vi "CRYOpen Edit Dialog.vi"(9 "List Index":i32, 10 "Stimulus In":T1={"StimulusType"="", "UseMLValArray"=[], "ML_axisArray"=[], "MLValLevelNameArray"=[], "Level(U)Array"=[1.0, 0.0, 0.0, 0.0, 0.0, 0.0, 0.26], "Start(Stop)FreqArray"=[20000.0, 20.0], "Start(Stop)AmpArray"=[0.5, 1.0], "StepResolutionArray"=[], "Unit_Array"=[], "DegValArray"=[], "DegUnitArray"=[], "Steps1"=19, "Cycle/step1(#)"=20, "Time/step1(s)"=0.01, "Transition1"=0.0, "SweepRate2"=1.0, "Freq3(Hz)"=0.0, "Steps3(#)"=19.0, "Cycles3(#)"=12, "StepSize3"=0.0, "wave time"="", "RMS_Value4"=0.0, "Peak_Value4"=0.0, "WavePath4"="", "RMS_unit4"="", "Peak_unit4"="", "wave Info"="", "dc_ctrl5_1"=0, "dc_ctrl5_2"=0, "dc_polar5"=0, "Max.Current"=0, "Steps5(#)"=19, "Time/Step5"=0.05, "Level5"=0.0, "StepsSize5Val"=0.0, "StepSize5Unit"="", "SweepType"=0, "Fixed/Ratio6"=0, "Transition6"=0.0, "Steps6(#)"=19.0, "Cycle/Steps6(#)"=12, "Time/Steps6(s)"=0.0, "Freq6(Hz)"=0.0, "Difference6(Hz)"=0.0, "Ratio6"="", "NoiseType7"=0, "Duration7(s)"=1.0, "MinFreq7(Hz)"=20000.0, "MaxFreq7(Hz)"=20.0, "MinFreq8(Hz)"=20000.0, "MaxFreq8(Hz)"=20.0, "FreqRounding8"=FALSE, "Duration8(s)"=1.0, "Tones8"=0.0, "RoundingVal8"=0.0, "ApplyEQ"=FALSE, "Duration(s)"=0.0, "CustomStimulusName "="", "Flatten Element Array"=[], "sine waves"=[], "Channel Out"=0, "RatioVal6"=0.0, "TabCtrl6"=enum."Master Tone", "Signal Type Name"="", "Help"="", "Channel Sel"=19, "V on DUT"=FALSE, "Output Imp"=6300.0, "Nominal Imp"=100.0} {"Nominal Imp" format="%.2p"; "Output Imp" format="%.2p"; "sine waves"."cycles" format="%.2f"; "sine waves"."ampl" format="%.2f"; "sine waves"."freq" format="%.2f"}) -> (1 "Ok Boolean":bool, 2 "Flatten Element Out":string, 3 "Stimulus Out":T1={"StimulusType"="", "UseMLValArray"=[], "ML_axisArray"=[], "MLValLevelNameArray"=[], "Level(U)Array"=[1.0, 0.0, 0.0, 0.0, 0.0, 0.0, 0.26], "Start(Stop)FreqArray"=[20000.0, 20.0], "Start(Stop)AmpArray"=[0.5, 1.0], "StepResolutionArray"=[], "Unit_Array"=[], "DegValArray"=[], "DegUnitArray"=[], "Steps1"=19, "Cycle/step1(#)"=20, "Time/step1(s)"=0.01, "Transition1"=0.0, "SweepRate2"=1.0, "Freq3(Hz)"=0.0, "Steps3(#)"=19.0, "Cycles3(#)"=12, "StepSize3"=0.0, "wave time"="", "RMS_Value4"=0.0, "Peak_Value4"=0.0, "WavePath4"="", "RMS_unit4"="", "Peak_unit4"="", "wave Info"="", "dc_ctrl5_1"=0, "dc_ctrl5_2"=0, "dc_polar5"=0, "Max.Current"=0, "Steps5(#)"=19, "Time/Step5"=0.05, "Level5"=0.0, "StepsSize5Val"=0.0, "StepSize5Unit"="", "SweepType"=0, "Fixed/Ratio6"=0, "Transition6"=0.0, "Steps6(#)"=19.0, "Cycle/Steps6(#)"=12, "Time/Steps6(s)"=0.0, "Freq6(Hz)"=0.0, "Difference6(Hz)"=0.0, "Ratio6"="", "NoiseType7"=0, "Duration7(s)"=1.0, "MinFreq7(Hz)"=20000.0, "MaxFreq7(Hz)"=20.0, "MinFreq8(Hz)"=20000.0, "MaxFreq8(Hz)"=20.0, "FreqRounding8"=FALSE, "Duration8(s)"=1.0, "Tones8"=0.0, "RoundingVal8"=0.0, "ApplyEQ"=FALSE, "Duration(s)"=0.0, "CustomStimulusName "="", "Flatten Element Array"=[], "sine waves"=[], "Channel Out"=0, "RatioVal6"=0.0, "TabCtrl6"=enum."Master Tone", "Signal Type Name"="", "Help"="", "Channel Sel"=19, "V on DUT"=FALSE, "Output Imp"=6300.0, "Nominal Imp"=100.0} {"Nominal Imp" format="%.2p"; "Output Imp" format="%.2p"; "sine waves"."cycles" format="%.2f"; "sine waves"."ampl" format="%.2f"; "sine waves"."freq" format="%.2f"})   [LabVIEW 2013]
uses:
  Typedef Control/CRYStimulus Cluster.ctl
  SubVI/CRYStimulus Global.vi
  Program/CRYRef nums global.vi
panel:
  # "(1,2,3,4,6_1,6_2,7,8)"
  # "(1,2,3,4,6_1,6_2,7,8)"
  # "(1,2,3,4,6_1,6_2,7,8)"
  # "(1,2,4,6_1,6_2,7,8)"
  # "(1,2,6)"
  # "(3,5)"
  # "(1,6,8)"
  # "(1,2,4,6_1,6_2,7,8)"
  # "(1,2,3,4,6_1,6_2,7,8)"
  # "(1,2,3,4,6_1,6_2,7,8)"
  # "(1,2,3,4,6_1,6_2,7,8)"
  # "(1,2,3,4,6_1,6_2,7,8)"
  # "(1,2,3,4,6_1,6_2,7,8)"
  # "(1,2,4,6_1,6_2,7,8)"
  # "(1,2,6)"
  # "(3,5)"
  # "(1,6,8)"
  # "(1,2,4,6_1,6_2,7,8)"
  # "(1,2,3,4,6_1,6_2,7,8)"
  # "(1,2,3,4,6_1,6_2,7,8)"
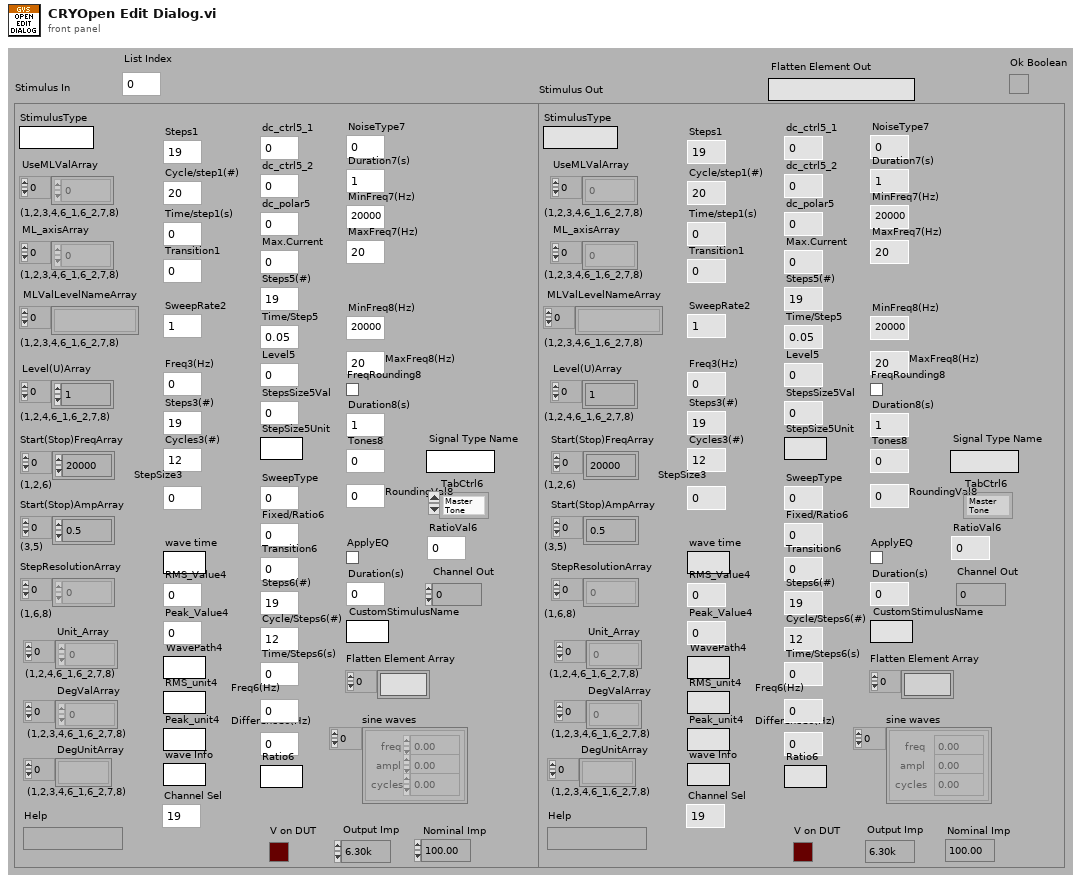
[diagram p1: front panel]
types:
  T1 = typedef "CRYStimulus Cluster.ctl" = cluster{"StimulusType":string, "UseMLValArray":u16[], "ML_axisArray":u16[], "MLValLevelNameArray":string[], "Level(U)Array":dbl[], "Start(Stop)FreqArray":dbl[], "Start(Stop)AmpArray":dbl[], "StepResolutionArray":u16[], "Unit_Array":u16[], "DegValArray":dbl[], "DegUnitArray":string[], "Steps1":i32, "Cycle/step1(#)":u32, "Time/step1(s)":dbl, "Transition1":dbl, "SweepRate2":dbl, "Freq3(Hz)":dbl, "Steps3(#)":dbl, "Cycles3(#)":u32, "StepSize3":dbl, "wave time":string, "RMS_Value4":dbl, "Peak_Value4":dbl, "WavePath4":string, "RMS_unit4":string, "Peak_unit4":string, "wave Info":string, "dc_ctrl5_1":u16, "dc_ctrl5_2":u16, "dc_polar5":u16, "Max.Current":u16, "Steps5(#)":u32, "Time/Step5":dbl, "Level5":dbl, "StepsSize5Val":dbl, "StepSize5Unit":string, "SweepType":u16, "Fixed/Ratio6":u16, "Transition6":dbl, "Steps6(#)":dbl, "Cycle/Steps6(#)":u32, "Time/Steps6(s)":dbl, "Freq6(Hz)":dbl, "Difference6(Hz)":dbl, "Ratio6":string, "NoiseType7":u16, "Duration7(s)":dbl, "MinFreq7(Hz)":dbl, "MaxFreq7(Hz)":dbl, "MinFreq8(Hz)":dbl, "MaxFreq8(Hz)":dbl, "FreqRounding8":bool, "Duration8(s)":dbl, "Tones8":dbl, "RoundingVal8":dbl, "ApplyEQ":bool, "Duration(s)":dbl, "CustomStimulusName ":string, "Flatten Element Array":string[], "sine waves":cluster{"freq":dbl, "ampl":dbl, "cycles":dbl}[], "Channel Out":i32, "RatioVal6":dbl, "TabCtrl6":enum32{"Master Tone", "Slave Tone"}, "Signal Type Name":string, "Help":string, "Channel Sel":u16, "V on DUT":bool, "Output Imp":dbl, "Nominal Imp":dbl}
  T2 = enum32{"Invalid", "Default", "Floating", "Floating/Auto-Hide", "Modal"}
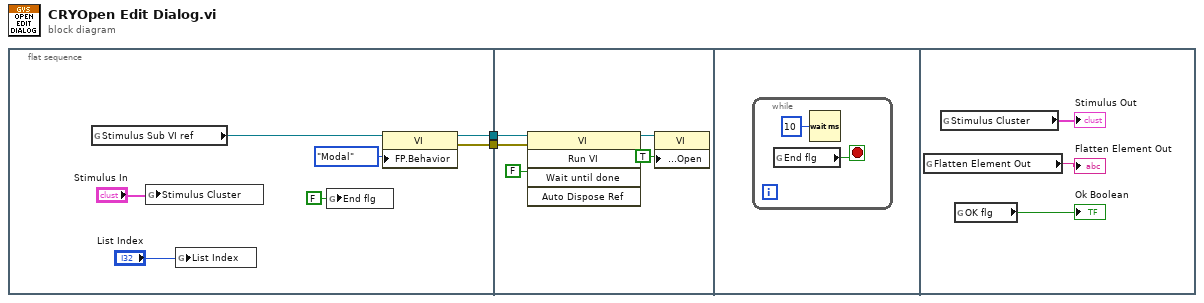
[diagram p0: block diagram]
diagram:
  n1 = flat-sequence {
    tunnel: [w9] -> w2
    tunnel: [w8] -> w1
    tunnel: w2 -> [w12]
    tunnel: w1 -> [w13]
    frame #0 {
      n2 = global read "CRYRef nums global.vi" "Stimulus Sub VI ref"() -> (w3:refnum<vi>)
      n3 = global write "CRYStimulus Global.vi" "Stimulus Cluster"("Stimulus In") -> ()
      n4 = global write "CRYStimulus Global.vi" "List Index"("List Index") -> ()
      n5 = global write "CRYStimulus Global.vi" "End flg"(FALSE ("End flg")) -> ()
      n6 = property class="VI"(reference=w3, "FP.Behavior"=T2."Modal" ("Front Panel Window:Behavior")) -> (reference out=w8:refnum<vi>, error out=w9:errorcluster)  [unwired: 1 in]
    }
    frame #1 {
      n7 = invoke class="VI" method="Run VI"(reference=w13, error in=w12, "Wait until done"=FALSE ("Wait Until Done")) -> (reference out=w10:refnum<vi>)  [unwired: 2 in, 4 out]
      n8 = property class="VI"(reference=w10, "Front Panel.Open"=TRUE ("Front Panel Window:Open")) -> ()  [unwired: 1 in, 2 out]
    }
    frame #2 {
      n9 = while {
        stop <- w16 stop-if-true
        n10 = global read "CRYStimulus Global.vi" "End flg"() -> (w16:bool)
        n11 = Wait (ms)(milliseconds to wait=u32 10) -> ()  [unwired: 1 out]
      }
    }
    frame #3 {
      n12 = global read "CRYStimulus Global.vi" "Flatten Element Out"() -> (→"Flatten Element Out":string)
      n13 = global read "CRYStimulus Global.vi" "Stimulus Cluster"() -> (→"Stimulus Out":T1)
      n14 = global read "CRYStimulus Global.vi" "OK flg"() -> (→"Ok Boolean":bool)
    }
  }
